vi "Curtin_Base64.vi"(8 "error in (no error)":errorcluster, 9 "String In":string, 11 "Base64 In":string) -> (0 "error out":errorcluster, 1 "Base64 Out":string, 3 "String Out":string)   [LabVIEW 2024]
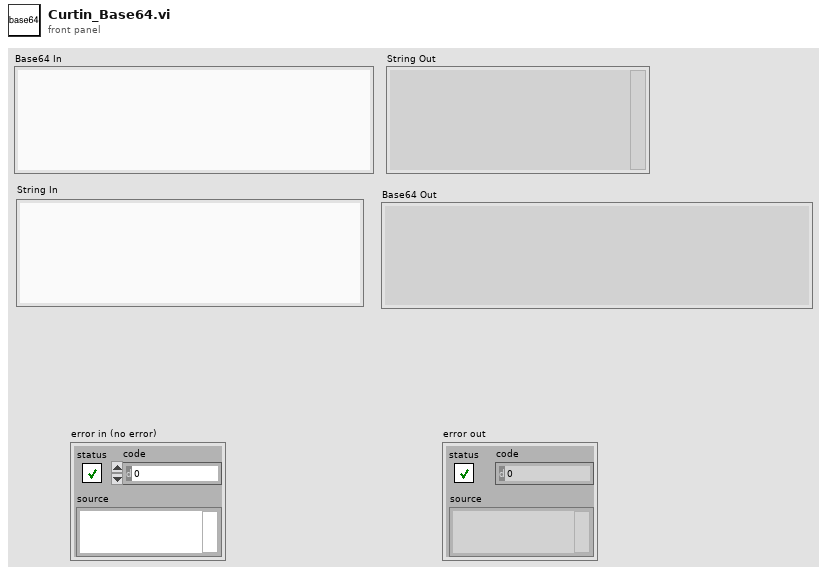
[diagram p1: front panel]
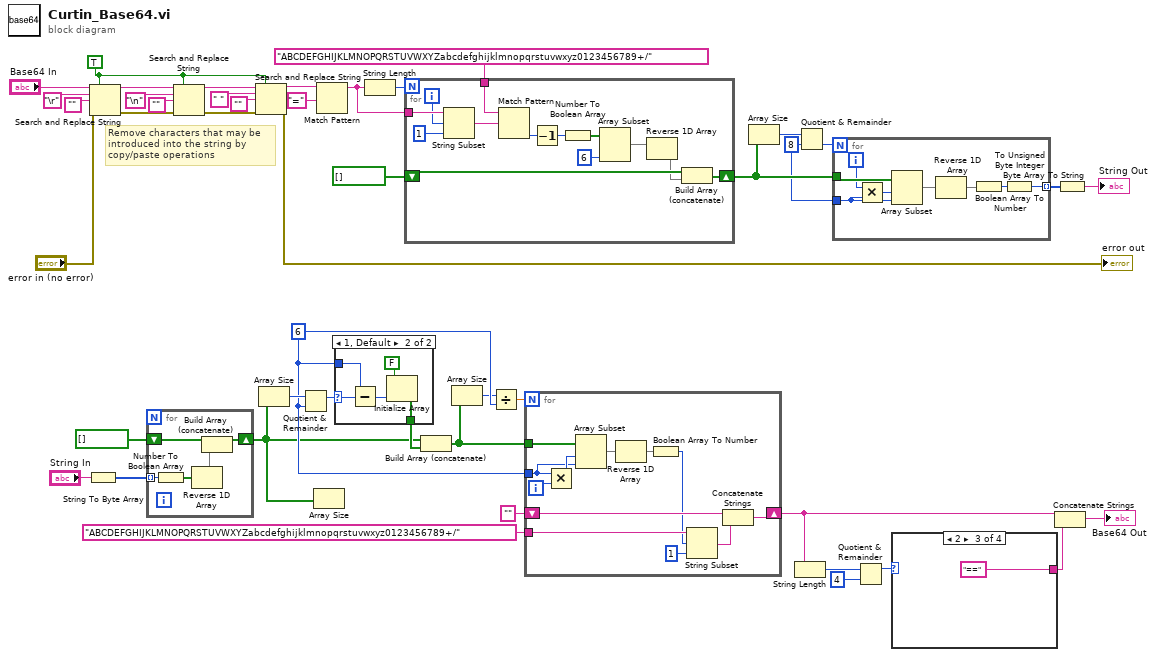
[diagram p0: block diagram]
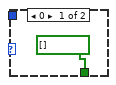
[diagram p2: hidden frame]
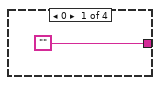
[diagram p3: hidden frame]
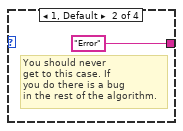
[diagram p4: hidden frame]
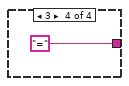
[diagram p5: hidden frame]
diagram:
  w4 = 6 ("y")
  w20 = TRUE ("replace all? (F)")
  w37 = 8 ("y")
  # "Remove characters that may be\nintroduced into the string by\ncopy/paste operations"
  n1 = String To Byte Array(string="String In") -> (unsigned byte array=w18:u8[])
  n2 = Search and Replace String(replace all?=w20, input string="Base64 In", search string="\r" ("replace string (\"\")"), replace string="", error in="error in (no error)") -> (result string=w30:string, error out=w28:errorcluster)  [unwired: 5 out]
  n3 = for {
    tunnel: w18 -> [w50] mode=indexing
    shift-right: [w47] -> w1
    shift-left: bool[] [] -> [w49]
    n4 = Number To Boolean Array(number=w50) -> (Boolean array=w48:bool[])
    n5 = Reverse 1D Array(array=w48) -> (reversed array=w46:bool[])
    n6 = Build Array (concatenate)(w49, w46) -> (w47:bool[])
  }
  n7 = Search and Replace String(replace all?=w20, input string=w30, search string="\n" ("replace string (\"\")"), replace string="", error in=w28) -> (result string=w24:string, error out=w23:errorcluster)  [unwired: 5 out]
  n8 = Search and Replace String(replace all?=w20, input string=w24, search string=" " ("replace string (\"\")"), replace string="", error in=w23) -> (result string=w21:string, error out=→"error out":errorcluster)  [unwired: 5 out]
  n9 = Array Size(array=w1) -> (size(s)=w7:i32)
  n10 = Quotient & Remainder(x=w7, y=w4) -> (x-y*floor(x/y)=w6:i32)  [unwired: 1 out]
  n11 = Array Size(array=w1) -> ()  [unwired: 1 out]
  n12 = Match Pattern(string=w21, regular expression="=") -> (before substring=w42:string)  [unwired: 4 out]
  n13 = case shown="1, Default" w6 {
    selector: w6 -> [_ w55]
    tunnel: [bool[] [] w52] -> w5
    tunnel: w4 -> [_ w54]
    frame 0 {
    }
    frame 1, Default {
      n14 = Subtract(x=w54, y=w55) -> (x-y=w56:i32)
      n15 = Initialize Array(FALSE, w56) -> (w52:bool[])
    }
  }
  n16 = String Length(string=w42) -> (length=w45:i32)
  n17 = for {
    N: w45 -> [_]
    tunnel: w42 -> [w69]
    tunnel: "ABCDEFGHIJKLMNOPQRSTUVWXYZabcdefghijklmnopqrstuvwxyz0123456789+/" -> [w66]
    shift-right: [w59] -> w38
    shift-left: bool[] [] -> [w58]
    i -> [w67]
    n18 = String Subset(string=w69, offset (0)=w67, length (rest)=1 ("length (rest)")) -> (substring=w65:string)
    n19 = Match Pattern(string=w66, regular expression=w65) -> (offset past match=w64:i32)  [unwired: 1 in, 3 out]
    n20 = Decrement(x=w64) -> (x-1=w63:i32)
    n21 = Number To Boolean Array(number=w63) -> (Boolean array=w62:bool[])
    n22 = Array Subset(array=w62, length=6) -> (w60:bool[])  [unwired: 1 in]
    n23 = Reverse 1D Array(array=w60) -> (reversed array=w57:bool[])
    n24 = Build Array (concatenate)(w58, w57) -> (w59:bool[])
  }
  n25 = Build Array (concatenate)(w1, w5) -> (w3:bool[])
  n26 = Array Size(array=w3) -> (size(s)=w2:i32)
  n27 = Divide(x=w2, y=w4) -> (x/y=w8:dbl)
  n28 = for {
    N: w8 -> [_]
    tunnel: w3 -> [w80]
    tunnel: w4 -> [w78]
    tunnel: "ABCDEFGHIJKLMNOPQRSTUVWXYZabcdefghijklmnopqrstuvwxyz0123456789+/" -> [w77]
    shift-right: [w75] -> w10
    shift-left: "" -> [w74]
    i -> [w81]
    n29 = Multiply(x=w78, y=w81) -> (x*y=w79:i32)
    n30 = Array Subset(array=w80, index=w79, length=w78) -> (w70:bool[])
    n31 = Reverse 1D Array(array=w70) -> (reversed array=w71:bool[])
    n32 = Boolean Array To Number(Boolean array=w71) -> (number=w72:u32)
    n33 = String Subset(string=w77, offset (0)=w72, length (rest)=1 ("length (rest)")) -> (substring=w73:string)
    n34 = Concatenate Strings(w74, w73) -> (w75:string)
  }
  n35 = Array Size(array=w38) -> (size(s)=w40:i32)
  n36 = String Length(string=w10) -> (length=w14:i32)
  n37 = Quotient & Remainder(x=w40, y=w37) -> (floor(x/y)=w39:i32)  [unwired: 1 out]
  n38 = for {
    N: w39 -> [_]
    tunnel: w38 -> [w89]
    tunnel: w37 -> [w88]
    tunnel: [w84] -> w36 mode=indexing
    i -> [w87]
    n39 = Multiply(x=w87, y=w88) -> (x*y=w82:i32)
    n40 = Array Subset(array=w89, index=w82, length=w88) -> (w86:bool[])
    n41 = Reverse 1D Array(array=w86) -> (reversed array=w83:bool[])
    n42 = Boolean Array To Number(Boolean array=w83) -> (number=w85:u32)
    n43 = To Unsigned Byte Integer(number=w85) -> (unsigned 8bit integer=w84:u8)
  }
  n44 = Quotient & Remainder(x=w14, y=4) -> (x-y*floor(x/y)=w12:i32)  [unwired: 1 out]
  n45 = case shown="2" w12 {
    tunnel: ["" "Error" "==" "="] -> w11
    frame 0 {
    }
    frame 1, Default {
      # "You should never\nget to this case. If\nyou do there is a bug\nin the rest of the algorithm."
    }
    frame 2 {
    }
    frame 3 {
    }
  }
  n46 = Concatenate Strings(w10, w11) -> (→"Base64 Out":string)
  n47 = Byte Array To String(unsigned byte array=w36) -> (string=→"String Out":string)
